vi "From Pythonic - Integer Array.vi"(4 "Pythonic Value":string) -> (1 "Integer Array":i64[](array[numeric]))   [LabVIEW 2012, in "OPI.lvclass"]
doc: "Convert pythonic values into LabVIEW data. This method can be helpfull to convert elements of tuples or dictionaries.\n\nReturn a 1D array of integer - LabVIEW I64 representation."
uses:
  OPI.lvclass
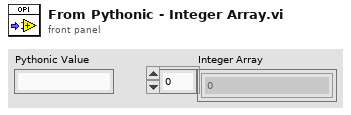
[diagram p1: front panel]
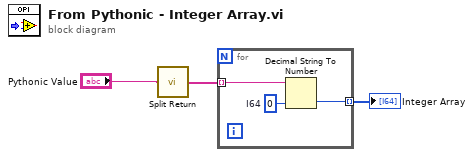
[diagram p0: block diagram]
diagram:
  n1 = call "Split Return.vi"("Return Value"="Pythonic Value") -> ("Split String"=w2:string[])
  n2 = for {
    tunnel: w2 -> [w6] mode=indexing
    tunnel: [w5] -> w3 mode=indexing
    w4 = i64 0  # I64
    n3 = Decimal String To Number(string=w6, default (0L)=w4) -> (number=w5:i64)  [unwired: 1 in, 1 out]
  }
  "Integer Array" <- w3
